vi "Measurement UI.vi"() -> ()   [LabVIEW 2021, in "IMD_Audio ADC_UI.lvlib"]
uses:
  IMD_Audio ADC_UI.lvlib
  shared/controls/PCM Interface Type_Copy.ctl
  <vilib>/PDM Acquisition Toolkit/shared/controls/Digital Edge.ctl
  shared/controls/Audio ADC Controls.lvlib
  <vilib>/PDM Acquisition Toolkit/shared/PDM Shared.lvlib
  shared/Audio ADC Shared.lvlib
panel:
  in  "MeasGraphs":T1(tab)
  out "FreqDomainGraph":cluster{"f0":dbl, "df":dbl, "Spectrum":dbl[]}(graph) caption="AC"
  out "TimeDomainGraph":waveform(dbl)(graph) caption="AC"
  out "dt":dbl
  out "t0":dbl
  out "df":dbl
  out "f0":dbl
  out "Time domain":dbl[](array[numeric])
  out "Spectrum":dbl[](array[numeric])
  out "IMD":dbl
  out "Channel":string
  in  "Victim channel resource name":string
  in  "Digital capture resource name":string
  out "MeasTable":string[][](table)
  in  "Configuration tab":enum32{"Protocol", "Measurement"}(tab)=enum."Measurement"
  in  "Endianness":enum32{"MSB First", "LSB First"}(ring)
  in  "Bit clock edge  sync":enum32{"Rising", "Falling"}(ring)=enum."Falling"
  in  "Frame sync edge for Channel 0":enum32{"Rising", "Falling"}(ring)=enum."Falling"
  in  "Channel count per frame":u32=2
  in  "Channel length":u32=32
  in  "Bit depth":u32=24
  in  "Channel 0 offset":u32=1
  in  "Data Justification":enum32{"Left Justified", "Right Justified"}(ring) caption="Data justification"
  in  "Frame length":u32=64
  in  "Frame sync pulse width":u32=32
  in  "I2S":bool
  in  "LJ":bool
  in  "RJ":bool
  in  "TDM":bool
  in  "Amplitude":dbl=-1.0 format="%#_pdB"
  in  "Amplitude ratio":dbl=1.0 format="%.1g"
  in  "High frequency":dbl=15000.0 format="%#_2pHz"
  in  "Low frequency":dbl=14000.0 format="%#_2pHz"
  in  "IMD standard":T2(ring)=enum."CCIF (11 kHz, 12 kHz, 1:1)"
  in  "Measurement Duration":dbl=0.1 caption="Measurement duration" format="%#_6ps"
  in  "Protocol capture resource name":string(combo) caption="Resource name"
  in  "Analog source resource name":string(combo) caption="Resource name"
  in  "Channel name":string
  in  "Full scale range":dbl=2.825 caption="FULL SCALE RANGE" format="%.3pV"
  in  "Data line":u32
  in  "Sample rate":dbl=192000.0 format="%#.6pHz"
  in  "Measurement settings":string="Measurement Settings"
  in  "Channel":u32
  in  "Analog source":string="Analog source"
  in  "Digital capture":string="Digital capture"
  # "Protocols"
  # "PCM data configuration"
  # "Frame sync clock control"
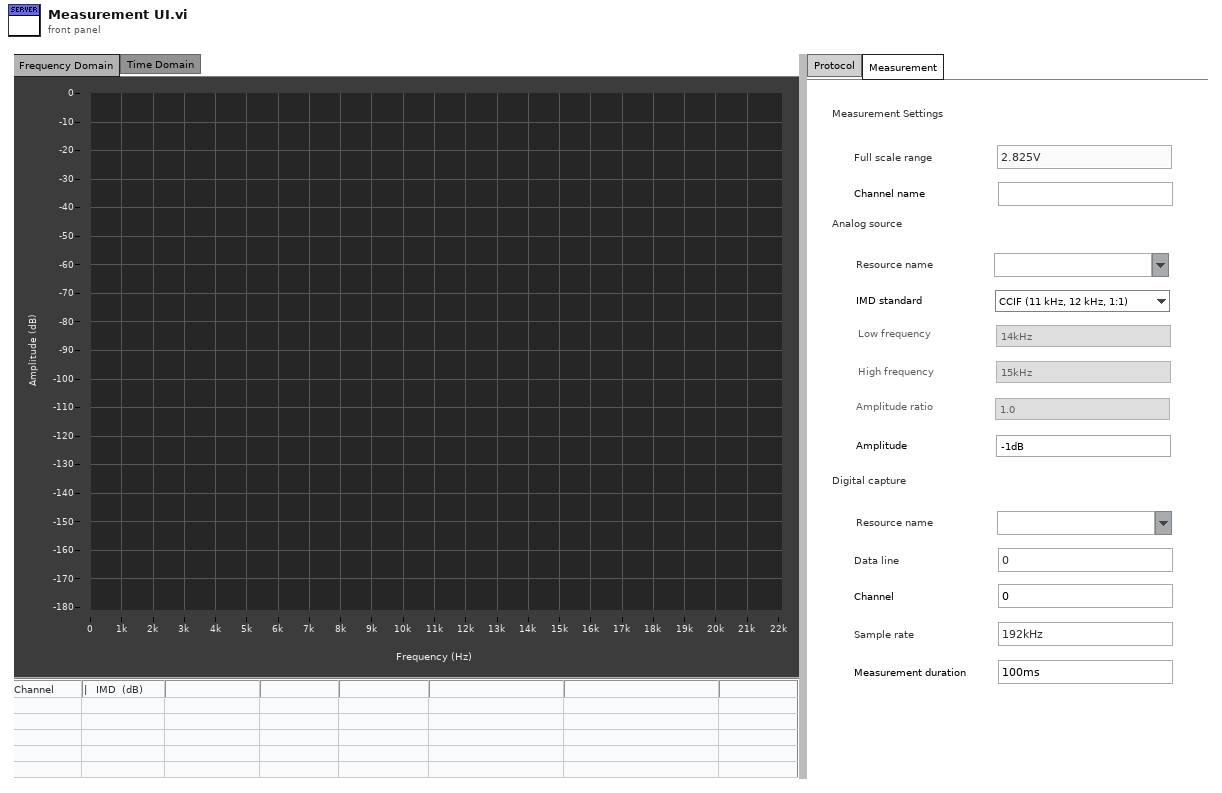
[diagram p1: front panel]
types:
  T1 = enum32{"Frequency Domain", "Time Domain", "Hidden Controls"}
  T2 = enum32{"SMPTE (60 Hz, 7000 Hz, 4:1)", "DIN (250 Hz, 8000 Hz, 4:1)", "CCIF (11 kHz, 12 kHz, 1:1)", "CCIF (19 kHz, 20 kHz, 1:1)", "Custom"}
  T3 = typedef "PDM Shared.lvlib/Digital Edge.ctl" = enum8{"Rising", "Falling"}
  T4 = typedef "Audio ADC Controls.lvlib/PCM Interface Type_Copy.ctl" = enum16{"I2S", "Left Justified", "Right Justified", "TDM 4 Channel", "TDM 6 Channel", "TDM 8 Channel", "DSP mode", "DSP mode with 1 bit delay", "PCM Short Frame", "PCM Long Frame"}
  T5 = enum8{"Enabled", "Disabled", "Disabled and Grayed Out"}
  T6 = typedef "PDM Shared.lvlib/PCM Frame Sync Control.ctl" = cluster{"Frame Length":u16, "Frame Sync Pulse Width":u16, "Bit Clock Edge  Sync":T3}
  T7 = typedef "PDM Shared.lvlib/PCM Data Format Configuration.ctl" = cluster{"Frame Sync Edge for Channel 0":T3, "Channel Count Per Frame":u8, "Channel Length":u16, "Bit Depth":u8, "Channel 0 Offset":u16, "Endianness":T8, "Data Justification":T9}
  T8 = typedef "PDM Shared.lvlib/PCM Bit Endianness.ctl" = enum16{"MSB First", "LSB First"}
  T9 = typedef "PDM Shared.lvlib/PCM Data Justification.ctl" = enum16{"Left Justified", "Right Justified"}
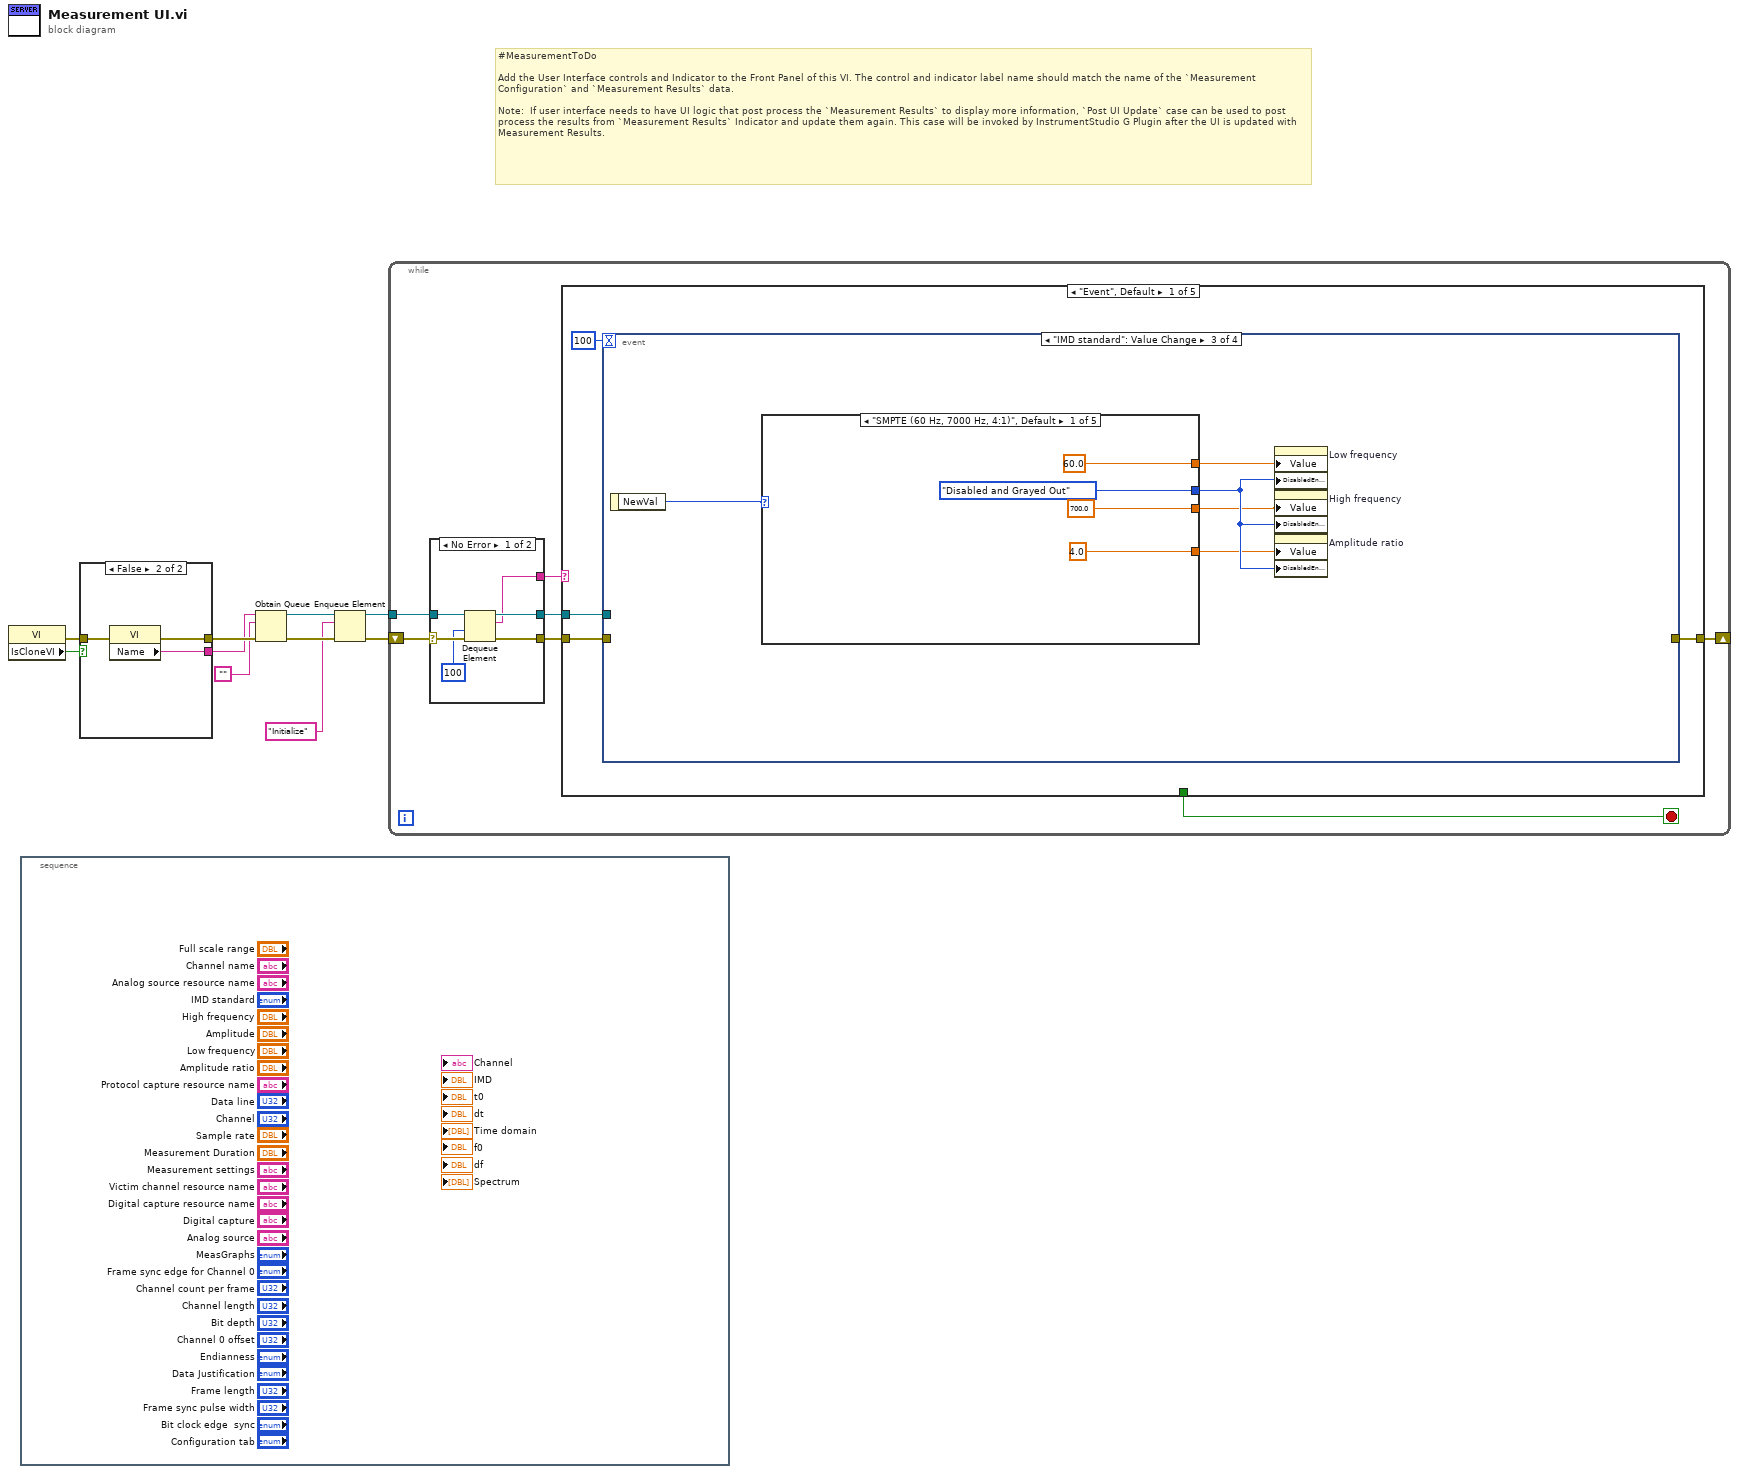
[diagram p0: block diagram]
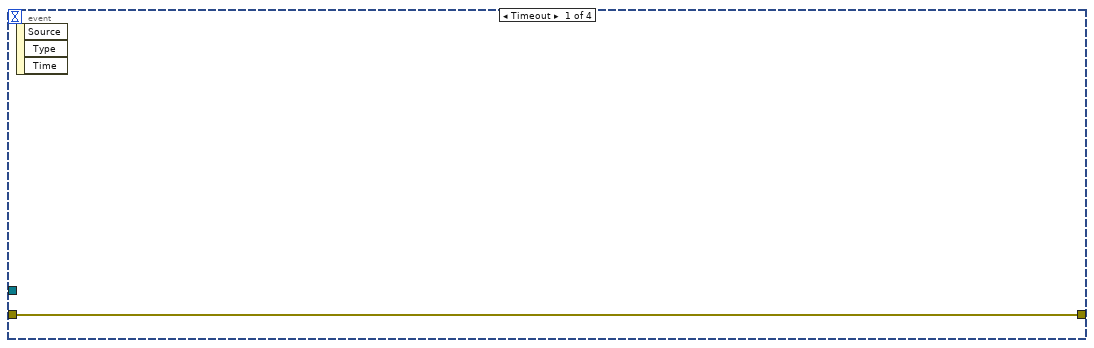
[diagram p2: hidden frame]
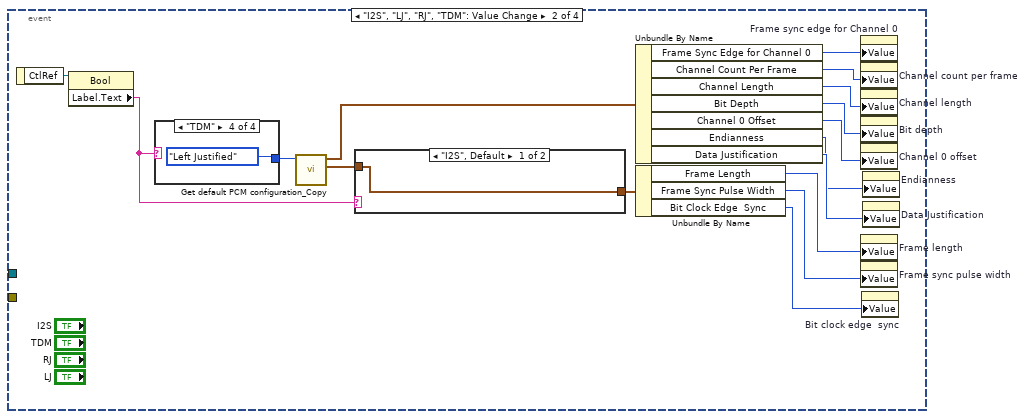
[diagram p3: hidden frame]
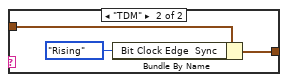
[diagram p4: hidden frame]
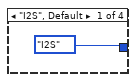
[diagram p5: hidden frame]
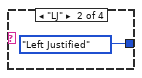
[diagram p6: hidden frame]
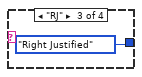
[diagram p7: hidden frame]
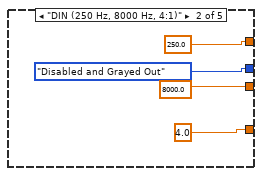
[diagram p8: hidden frame]
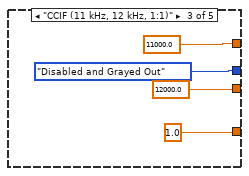
[diagram p9: hidden frame]
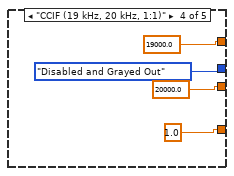
[diagram p10: hidden frame]
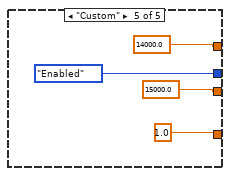
[diagram p11: hidden frame]
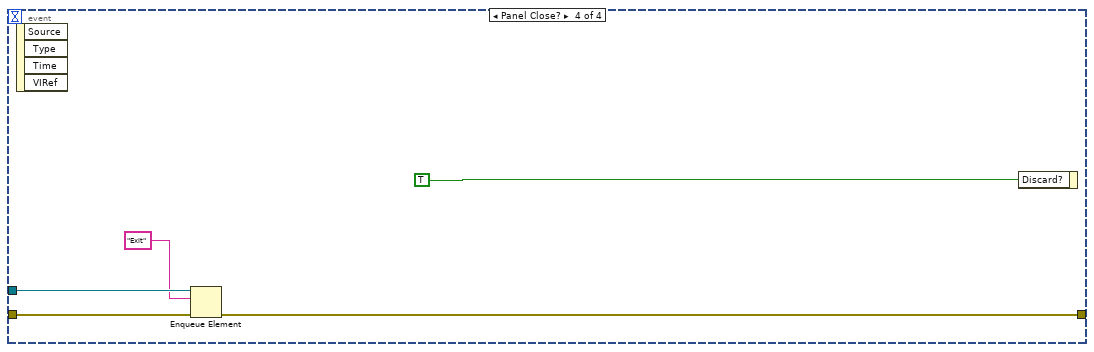
[diagram p12: hidden frame]
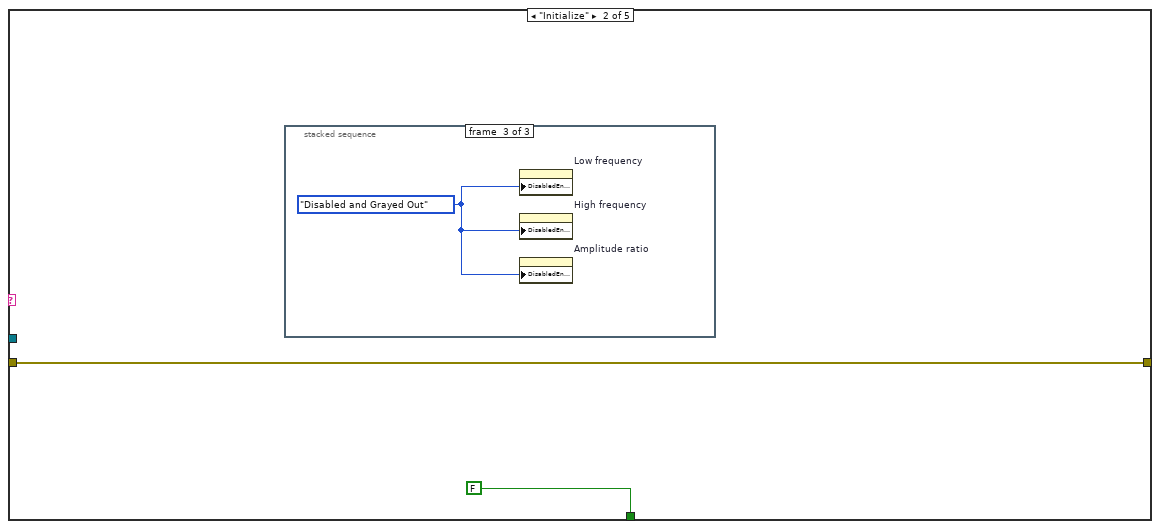
[diagram p13: hidden frame]
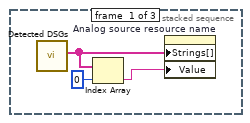
[diagram p14: hidden frame]
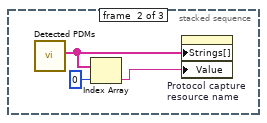
[diagram p15: hidden frame]
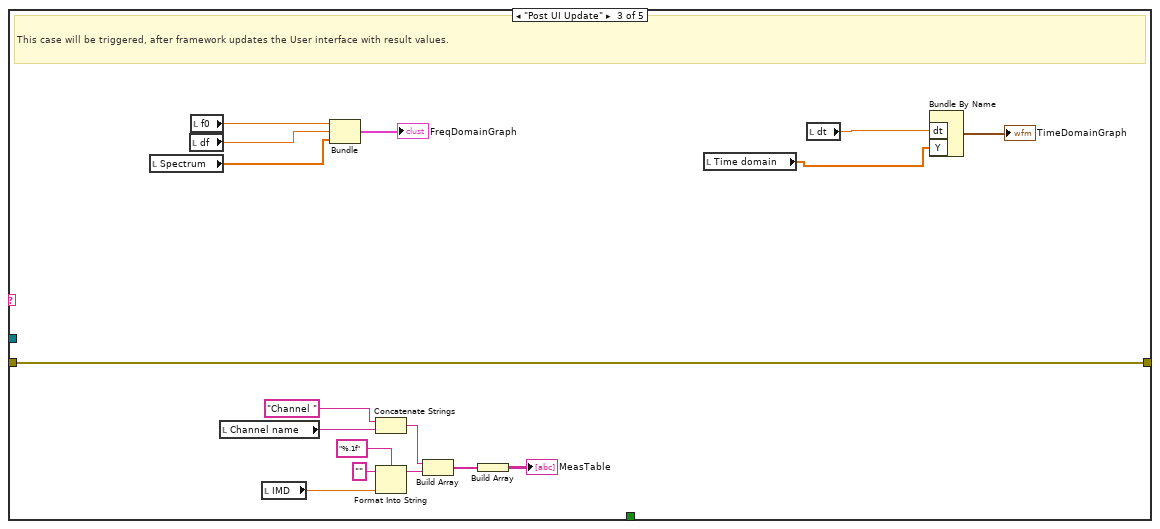
[diagram p16: hidden frame]
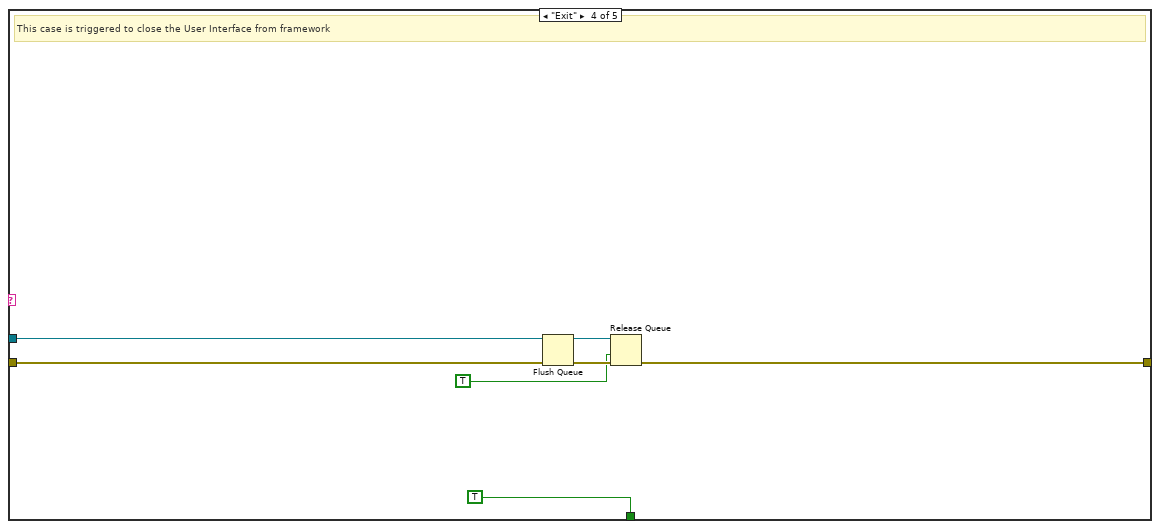
[diagram p17: hidden frame]
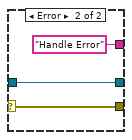
[diagram p19: hidden frame]
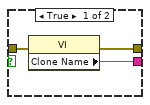
[diagram p20: hidden frame]
diagram:
  # "#MeasurementToDo  \n\nAdd the User Interface controls and Indicator to the Front Panel of this VI. The control and indicator label name should match the name of the `Measurement Configuration` and `Measurement Results` data.\n\nNote:  If user interface needs to have UI logic that post process the `Measurement Results` to display more information, `Post UI Update` case can be used to post process the results from `Measurement Results` Indicator and update them again. This case will be invoked by InstrumentStudio G Plugin after the UI is updated with Measurement Results."
  n1 = property class="VI"() -> (error out=w1:errorcluster, "IsCloneVI"=w2:bool)  [unwired: 2 in, 1 out]
  n2 = stacked-sequence {
    frame #0 {
    }
  }
  n3 = case shown="False" w2 {
    tunnel: [w13 w16] -> w10
    tunnel: [w12 w15] -> w9
    tunnel: w1 -> [w11 w14]
    frame True {
      n4 = property class="VI"(error in=w11) -> (error out=w13:errorcluster, "Clone Name"=w12:string)  [unwired: 1 in, 1 out]
    }
    frame False {
      n5 = property class="VI"(error in=w14) -> (error out=w16:errorcluster, "Name"=w15:string)  [unwired: 1 in, 1 out]
    }
  }
  n6 = Obtain Queue(name (unnamed)=w9, element data type="", error in (no error)=w10) -> (queue out=w6:refnum<queue>, error out=w8:errorcluster)  [unwired: 2 in, 1 out]
  n7 = Enqueue Element(queue=w6, element="Initialize", error in (no error)=w8) -> (queue out=w5:refnum<queue>, error out=w7:errorcluster)  [unwired: 1 in, 1 out]
  n8 = while {
    shift-right: [w18] -> _
    shift-left: w7 -> [w23]
    tunnel: w5 -> [w21]
    stop <- w17 stop-if-true
    n9 = case shown="No Error" w23 {
      selector: w23 -> [w122 w125]
      tunnel: [w121 w125] -> w22
      tunnel: w21 -> [w120 w124]
      tunnel: [w119 w124] -> w20
      tunnel: [w118 "Handle Error"] -> w19
      frame No Error {
        n10 = Dequeue Element(queue=w120, timeout in ms (-1)=100, error in (no error)=w122) -> (queue out=w119:refnum<queue>, element=w118:string, error out=w121:errorcluster)  [unwired: 1 out]
      }
      frame Error {
      }
    }
    n11 = case shown="\"Event\", Default" w19 {
      tunnel: w22 -> [w26 w84 w103 w115 w116]
      tunnel: w20 -> [w24 _ _ w113 _]
      tunnel: [w27 w84 w103 w110 w116] -> w18
      tunnel: [_ FALSE _ TRUE _] -> w17
      frame "Event", Default {
        n12 = event shown="[2] \"IMD standard\": Value Change" {
          selector: _ -> [_ _ _ _]
          dyn-events: _ -> [_ _ _ _]
          timeout: 100 -> [_ _ _ _]
          tunnel: [w28 _ _ w80] -> w27
          tunnel: w26 -> [w28 _ _ w81]
          tunnel: w24 -> [_ _ _ w79]
          event Timeout {
            n13 = event-data() -> ()  [unwired: 1 in, 3 out]
          }
          event "I2S", "LJ", "RJ", "TDM": Value Change {
            n14 = event-data() -> ("CtlRef"=w44:refnum<vi>)  [unwired: 1 in]
            n15 = property class="Bool"(reference=w44) -> ("Label.Text"=w43:string)  [unwired: 1 in, 2 out]
            n16 = case shown="\"TDM\"" w43 {
              tunnel: [PCM_Interface_Type_Copy."I2S" ("PCM Interfaces") PCM_Interface_Type_Copy."Left Justified" ("PCM Interfaces") PCM_Interface_Type_Copy."Right Justified" ("PCM Interfaces") PCM_Interface_Type_Copy."Left Justified" ("PCM Interfaces")] -> w33
              frame "I2S", Default {
              }
              frame "LJ" {
              }
              frame "RJ" {
              }
              frame "TDM" {
              }
            }
            n17 = call "Get default PCM configuration_Copy.vi"("PCM Interfaces"=w33) -> ("Frame Sync Clock Control"=w31:T6, "PCM Data Configuration"=w32:T7)  [unwired: 9 in]
            n18 = case shown="\"I2S\", Default" w43 {
              tunnel: [w45 w47] -> w42
              tunnel: w31 -> [w45 w46]
              frame "I2S", Default {
              }
              frame "TDM" {
                n19 = Bundle By Name(cluster=w46, "Bit Clock Edge  Sync"=Digital_Edge."Rising") -> (w47:T6)
              }
            }
            n20 = Unbundle By Name(w32) -> ("Frame Sync Edge for Channel 0"=w41:T3, "Channel Count Per Frame"=w40:u8, "Channel Length"=w39:u16, "Bit Depth"=w38:u8, "Channel 0 Offset"=w37:u16, "Endianness"=w29:T8, "Data Justification"=w34:T9)
            n21 = Unbundle By Name(w42) -> ("Frame Length"=w36:u16, "Frame Sync Pulse Width"=w35:u16, "Bit Clock Edge  Sync"=w30:T3)
            n22 = property on="Frame sync edge for Channel 0" class="Enum (strict)"("Value"=w41) -> ()  [unwired: 2 in, 2 out]
            n23 = property on="Channel count per frame" class="DigNum (strict)"("Value"=w40) -> ()  [unwired: 2 in, 2 out]
            n24 = property on="Channel length" class="DigNum (strict)"("Value"=w39) -> ()  [unwired: 2 in, 2 out]
            n25 = property on="Bit depth" class="DigNum (strict)"("Value"=w38) -> ()  [unwired: 2 in, 2 out]
            n26 = property on="Channel 0 offset" class="DigNum (strict)"("Value"=w37) -> ()  [unwired: 2 in, 2 out]
            n27 = property on="Frame length" class="DigNum (strict)"("Value"=w36) -> ()  [unwired: 2 in, 2 out]
            n28 = property on="Frame sync pulse width" class="DigNum (strict)"("Value"=w35) -> ()  [unwired: 2 in, 2 out]
            n29 = property on="Bit clock edge  sync" class="Enum (strict)"("Value"=w30) -> ()  [unwired: 2 in, 2 out]
            n30 = property on="Endianness" class="Enum (strict)"("Value"=w29) -> ()  [unwired: 2 in, 2 out]
            n31 = property on="Data Justification" class="Enum (strict)"("Value"=w34) -> ()  [unwired: 2 in, 2 out]
          }
          event "IMD standard": Value Change {
            n32 = event-data() -> ("NewVal"=w57:T2)  [unwired: 1 in]
            n33 = case shown="\"SMPTE (60 Hz, 7000 Hz, 4:1)\", Default" w57 {
              tunnel: [60.0 ("Low frequency") 250.0 ("Low frequency") 11000.0 ("Low frequency") 19000.0 ("Low frequency") 14000.0 ("Low frequency")] -> w56
              tunnel: [T5."Disabled and Grayed Out" ("Disabled") T5."Disabled and Grayed Out" ("Disabled") T5."Disabled and Grayed Out" ("Disabled") T5."Disabled and Grayed Out" ("Disabled") T5."Enabled" ("Disabled")] -> w55
              tunnel: [700.0 ("Low frequency") 8000.0 ("Low frequency") 12000.0 ("Low frequency") 20000.0 ("Low frequency") 15000.0 ("Low frequency")] -> w54
              tunnel: [4.0 ("Low frequency") 4.0 ("Low frequency") 1.0 ("Low frequency") 1.0 ("Low frequency") 1.0 ("Low frequency")] -> w53
              frame "SMPTE (60 Hz, 7000 Hz, 4:1)", Default {
              }
              frame "DIN (250 Hz, 8000 Hz, 4:1)" {
              }
              frame "CCIF (11 kHz, 12 kHz, 1:1)" {
              }
              frame "CCIF (19 kHz, 20 kHz, 1:1)" {
              }
              frame "Custom" {
              }
            }
            n34 = property on="Low frequency" class="DigNum (strict)"("Value"=w56, "DisabledEnum"=w55) -> ()  [unwired: 2 in, 2 out]
            n35 = property on="High frequency" class="DigNum (strict)"("Value"=w54, "DisabledEnum"=w55) -> ()  [unwired: 2 in, 2 out]
            n36 = property on="Amplitude ratio" class="DigNum (strict)"("Value"=w53, "DisabledEnum"=w55) -> ()  [unwired: 2 in, 2 out]
          }
          event Panel Close? {
            n37 = event-data() -> ()  [unwired: 1 in, 4 out]
            n38 = Enqueue Element(queue=w79, element="Exit", error in (no error)=w81) -> (error out=w80:errorcluster)  [unwired: 1 in, 2 out]
            n39 = event-data("Discard?"=TRUE) -> ()  [unwired: 1 in, 1 out]
          }
        }
      }
      frame "Initialize" {
        n40 = stacked-sequence {
          frame #0 {
            n41 = call "Detected DSGs.vi"() -> ("AO channels"=w87:string[])  [unwired: 11 in]
            n42 = Index Array(array=w87, index=0) -> (element=w86:string)
            n43 = property on="Analog source resource name" class="CmbBox"("Strings[]"=w87, "Value"=w86) -> ()  [unwired: 2 in, 2 out]
          }
          frame #1 {
            n44 = call "Detected PDMs.vi"() -> ("PDM devices"=w89:string[])  [unwired: 11 in]
            n45 = Index Array(array=w89, index=0) -> (element=w88:string)
            n46 = property on="Protocol capture resource name" class="CmbBox"("Strings[]"=w89, "Value"=w88) -> ()  [unwired: 2 in, 2 out]
          }
          frame #2 {
            w91 = T5."Disabled and Grayed Out" ("Disabled")
            n47 = property on="Low frequency" class="DigNum (strict)"("DisabledEnum"=w91) -> ()  [unwired: 2 in, 2 out]
            n48 = property on="High frequency" class="DigNum (strict)"("DisabledEnum"=w91) -> ()  [unwired: 2 in, 2 out]
            n49 = property on="Amplitude ratio" class="DigNum (strict)"("DisabledEnum"=w91) -> ()  [unwired: 2 in, 2 out]
          }
        }
      }
      frame "Post UI Update" {
        # "This case will be triggered, after framework updates the User interface with result values."
        n50 = local read "Spectrum"() -> (w97:dbl[])
        n51 = local read "df"() -> (w100:dbl)
        n52 = local read "f0"() -> (w101:dbl)
        n53 = local read "Channel name"() -> (w94:string)
        n54 = local read "IMD"() -> (w102:dbl)
        n55 = Bundle("f0"=w101, "df"=w100, "Spectrum"=w97) -> (→"FreqDomainGraph":cluster{"f0":dbl, "df":dbl, "Spectrum":dbl[]})  [unwired: 1 in]
        n56 = Concatenate Strings("Channel " ("string"), w94) -> (w93:string)
        n57 = Format Into String(format string="%.1f", initial string="", w102) -> (resulting string=w106:string)  [unwired: 1 in, 1 out]
        n58 = Build Array(w93, w106) -> (w105:string[])
        n59 = Build Array(w105) -> (→"MeasTable":string[][])
        n60 = local read "Time domain"() -> (w95:dbl[])
        n61 = local read "dt"() -> (w98:dbl)
        n62 = Bundle By Name("dt"=w98, "Y"=w95) -> (→"TimeDomainGraph":waveform(dbl))  [unwired: 1 in]
      }
      frame "Exit" {
        # "This case is triggered to close the User Interface from framework"
        n63 = Flush Queue(queue=w113, error in (no error)=w115) -> (queue out=w112:refnum<queue>, error out=w111:errorcluster)  [unwired: 1 out]
        n64 = Release Queue(queue=w112, force destroy? (F)=TRUE, error in (no error)=w111) -> (error out=w110:errorcluster)  [unwired: 2 out]
      }
      frame "Handle Error" {
      }
    }
  }
